vi "Filter Only.vi"(7 "Bookmark":T1, 8 "Error In":errorcluster, 11 "VI Bookmarks":T2[](array[typedef])) -> (0 "Error Out":errorcluster, 3 "Graves":T2[](array[typedef]))   [LabVIEW 2017, in "Bookmark Manager.lvlib"]
doc: "Filters out all bookmarks that are NOT graves"
uses:
  Bookmark Manager.lvlib
  VI Bookmark.ctl
  VI Information.ctl
  Application Information.ctl
  Eulogy/Public/Typedefs/Bookmarks.ctl
  Eulogy/Eulogy.lvlib
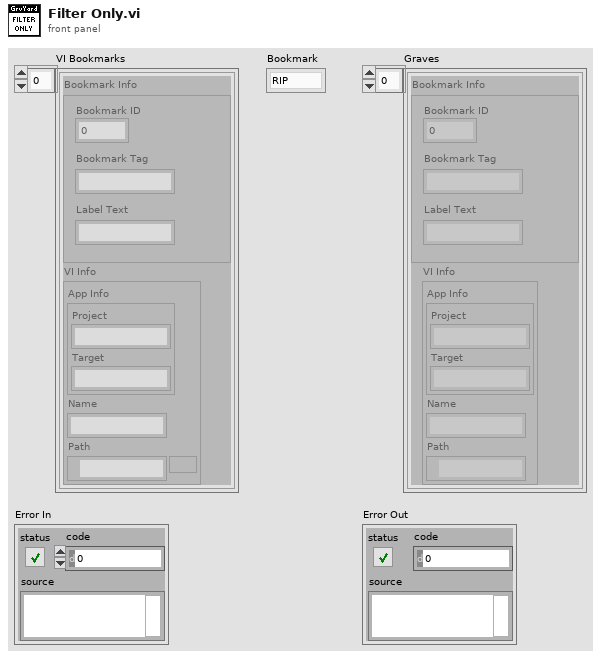
[diagram p1: front panel]
types:
  T1 = typedef "Eulogy.lvlib/Bookmarks.ctl" = enum16{"RIP", "Zombie"}
  T2 = typedef "Bookmark Manager.lvlib/VI Bookmark.ctl" = cluster{"Bookmark Info":cluster{"Bookmark ID":u32, "Bookmark Tag":string, "Label Text":string}, "VI Info":T3}
  T3 = typedef "Bookmark Manager.lvlib/VI Information.ctl" = cluster{"App Info":T4, "Name":string, "Path":path}
  T4 = typedef "Bookmark Manager.lvlib/Application Information.ctl" = cluster{"Project":string, "Target":string}
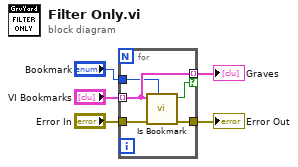
[diagram p0: block diagram]
diagram:
  n1 = for {
    tunnel: [w9] -> w2 mode=indexing if=w10
    tunnel: "Error In" -> [w8]
    tunnel: [w7] -> w4
    tunnel: "VI Bookmarks" -> [w9] mode=indexing
    tunnel: "Bookmark" -> [w6]
    n2 = call "Is Bookmark.vi"("Bookmark"=w6, "Error In"=w8, "VI Bookmark"=w9) -> ("Error Out"=w7:errorcluster, "Is Bookmark"=w10:bool)  [unwired: 7 in]
  }
  "Error Out" <- w4
  "Graves" <- w2
